vi "Read demandRotRaDec.vi"(8 "error in (no error)":errorcluster, 11 "NewScienceTarget in":refnum<class "NewScienceTarget.lvclass">) -> (0 "error out":errorcluster, 2 "RADecParameters.lvclass":refnum<class "RADecParameters.lvclass">, 3 "NewScienceTarget out":refnum<class "NewScienceTarget.lvclass">)   [LabVIEW 2022 SP3, in "TCSDataDefinitions.lvlib" / "TCSPublicStatus.lvlib" / "NewScienceTarget.lvclass"]
uses:
  NewScienceTarget.lvclass
  TCSCommand/TargetConfiguration/Target/FixedTarget/RADecParameters/RADecParameters.lvclass
  NewScienceTarget.lvclass/NewScienceTarget.ctl
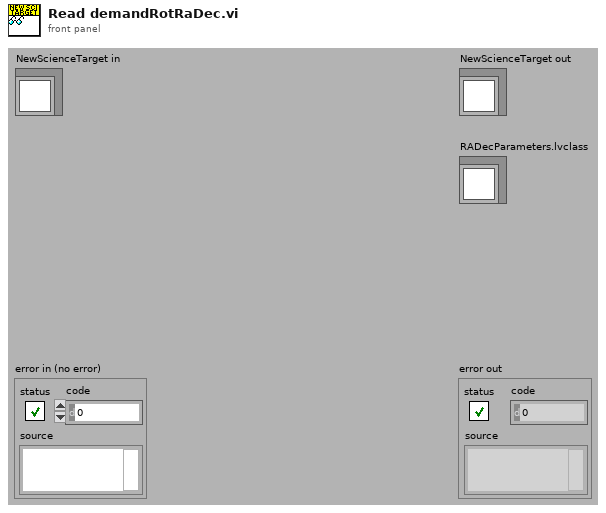
[diagram p1: front panel]
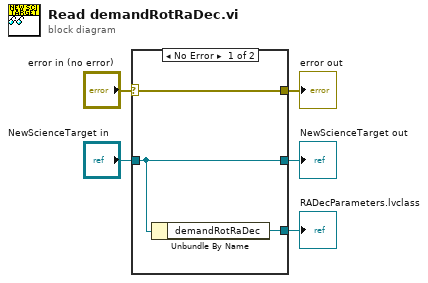
[diagram p0: block diagram]
diagram:
  n1 = case shown="No Error" "error in (no error)" {
    selector: "error in (no error)" -> [w8 w9]
    tunnel: [w8 w9] -> w4
    tunnel: [w7 w10] -> w2
    tunnel: "NewScienceTarget in" -> [w7 w10]
    tunnel: [w6 _] -> w1
    frame No Error {
      n2 = Unbundle By Name(w7) -> ("demandRotRaDec"=w6:refnum<class "RADecParameters.lvclass">)
    }
    frame Error {
    }
  }
  "error out" <- w4
  "NewScienceTarget out" <- w2
  "RADecParameters.lvclass" <- w1
